vi "SInusoidy.vi"() -> ()   [LabVIEW 2020]
panel:
  in  "Amplituda 16":dbl
  in  "Faza 16":dbl
  in  "k 16":dbl
  in  "N 16":i32
  in  "Amplituda 15":dbl
  in  "Faza 15":dbl
  in  "k 15":dbl
  in  "N 15":i32
  out "Trzy osatatnie figury":cluster{"Array":dbl[], "Array":dbl[]}[](graph)
  in  "Amplituda 14":dbl
  in  "Faza 14":dbl
  in  "k 14":dbl
  in  "N 14":i32
  in  "Amplituda 13":dbl
  in  "Faza 13":dbl
  in  "k 13":dbl
  in  "N 13":i32
  in  "Amplituda 12":dbl
  in  "Faza 12":dbl
  in  "k 12":dbl
  in  "N 12":i32
  in  "Amplituda 11":dbl
  in  "Faza 11":dbl
  in  "k 11":dbl
  in  "N 11":i32
  in  "Amplituda 10":dbl
  in  "Faza 10":dbl
  in  "k 10":dbl
  in  "N 10":i32
  in  "Amplituda 9":dbl
  in  "Faza 9":dbl
  in  "k 9":dbl
  in  "N 9":i32
  in  "Amplituda 8":dbl
  in  "Faza 8":dbl
  in  "k 8":dbl
  in  "N 8":i32
  in  "Amplituda 7":dbl
  in  "Faza 7":dbl
  in  "k 7":dbl
  in  "N 7":i32
  out "Trzy pierwsze figury Lissajous":cluster{"Array":dbl[], "Array":dbl[]}[](graph)
  in  "Amplituda 6":dbl
  in  "Faza 6":dbl
  in  "k 6":dbl
  in  "N 6":i32
  in  "Amplituda 5":dbl
  in  "Faza 5":dbl
  in  "k 5":dbl
  in  "N 5":i32
  out "Dowolne figury Lissajous":cluster{"Y":dbl[], "Y":dbl[]}[](graph)
  in  "Amplituda 4":dbl
  in  "Faza 4":dbl
  in  "k 4":dbl
  in  "N 4":i32
  in  "Amplituda 3":dbl
  in  "Faza 3":dbl
  in  "k 3":dbl
  in  "N 3":i32
  in  "Amplituda 2":dbl
  in  "Faza 2":dbl
  in  "k 2":dbl
  in  "N 2":i32
  out "Do cosinusa":dbl[](graph)
  out "Do sinusa":dbl[](graph)
  in  "N":i32
  in  "Amplituda":dbl
  in  "Faza":dbl
  in  "k":dbl
  # "Pierwsza figura"
  # "Druga figura"
  # "Trzecia Figura"
  # "Do ostatnich figur"
  # "uno"
  # "duo"
  # "tres"
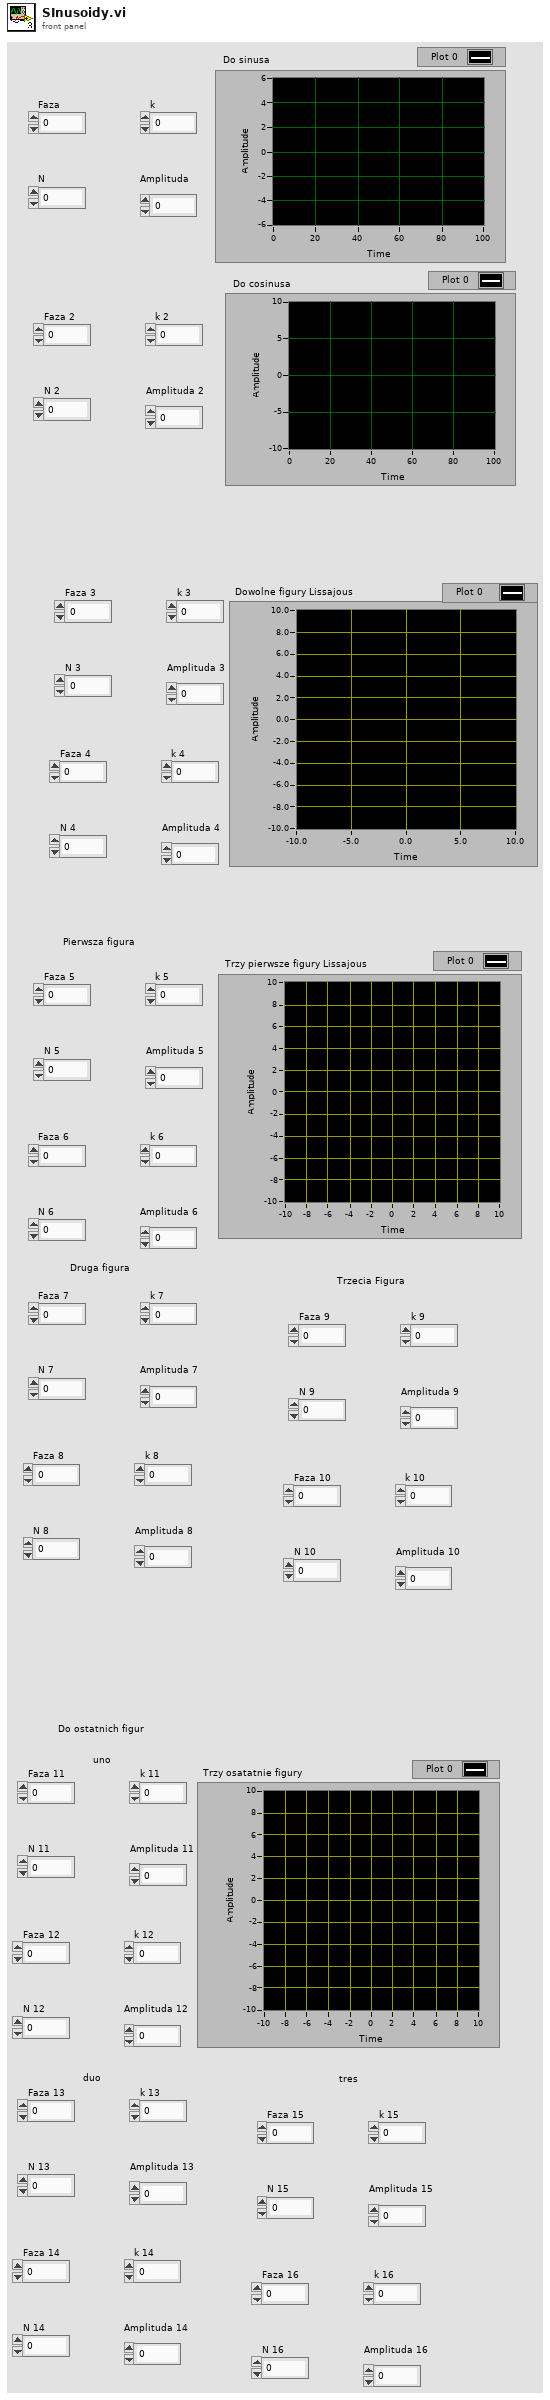
[diagram p1: front panel]
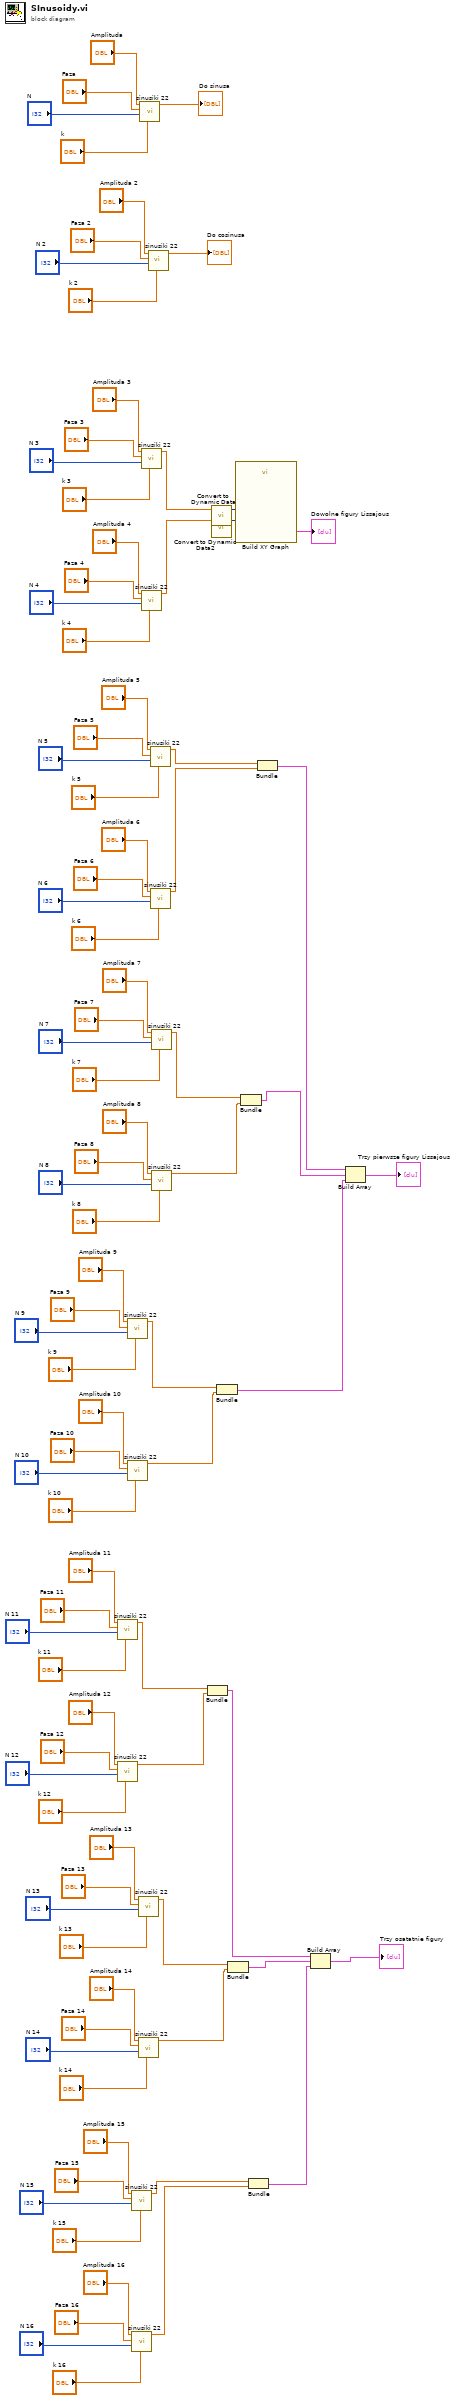
[diagram p0: block diagram]
diagram:
  n1 = call "sinusiki 22.vi"("k"="k 11", "N"="N 11", "Faza"="Faza 11", "Amplituda"="Amplituda 11") -> ("Array"=w26:dbl[])  [unwired: 7 in]
  n2 = call "sinusiki 22.vi"("k"="k 12", "N"="N 12", "Faza"="Faza 12", "Amplituda"="Amplituda 12") -> ("Array"=w25:dbl[])  [unwired: 7 in]
  n3 = call "sinusiki 22.vi"("k"="k 9", "N"="N 9", "Faza"="Faza 9", "Amplituda"="Amplituda 9") -> ("Array"=w38:dbl[])  [unwired: 7 in]
  n4 = call "sinusiki 22.vi"("k"="k 10", "N"="N 10", "Faza"="Faza 10", "Amplituda"="Amplituda 10") -> ("Array"=w37:dbl[])  [unwired: 7 in]
  n5 = call "sinusiki 22.vi"("k"="k 15", "N"="N 15", "Faza"="Faza 15", "Amplituda"="Amplituda 15") -> ("Array"=w3:dbl[])  [unwired: 7 in]
  n6 = call "sinusiki 22.vi"("k"="k 16", "N"="N 16", "Faza"="Faza 16", "Amplituda"="Amplituda 16") -> ("Array"=w2:dbl[])  [unwired: 7 in]
  n7 = call "sinusiki 22.vi"("k"="k 13", "N"="N 13", "Faza"="Faza 13", "Amplituda"="Amplituda 13") -> ("Array"=w16:dbl[])  [unwired: 7 in]
  n8 = call "sinusiki 22.vi"("k"="k 14", "N"="N 14", "Faza"="Faza 14", "Amplituda"="Amplituda 14") -> ("Array"=w15:dbl[])  [unwired: 7 in]
  n9 = call "sinusiki 22.vi"("k"="k", "N"="N", "Faza"="Faza", "Amplituda"="Amplituda") -> ("Array"=→"Do sinusa":dbl[])  [unwired: 7 in]
  n10 = call "sinusiki 22.vi"("k"="k 3", "N"="N 3", "Faza"="Faza 3", "Amplituda"="Amplituda 3") -> ("Array"=w72:dbl[])  [unwired: 7 in]
  n11 = call "sinusiki 22.vi"("k"="k 4", "N"="N 4", "Faza"="Faza 4", "Amplituda"="Amplituda 4") -> ("Array"=w70:dbl[])  [unwired: 7 in]
  n12 = call "sinusiki 22.vi"("k"="k 2", "N"="N 2", "Faza"="Faza 2", "Amplituda"="Amplituda 2") -> ("Array"=→"Do cosinusa":dbl[])  [unwired: 7 in]
  n13 = call "sinusiki 22.vi"("k"="k 5", "N"="N 5", "Faza"="Faza 5", "Amplituda"="Amplituda 5") -> ("Array"=w60:dbl[])  [unwired: 7 in]
  n14 = call "sinusiki 22.vi"("k"="k 6", "N"="N 6", "Faza"="Faza 6", "Amplituda"="Amplituda 6") -> ("Array"=w59:dbl[])  [unwired: 7 in]
  n15 = call "sinusiki 22.vi"("k"="k 7", "N"="N 7", "Faza"="Faza 7", "Amplituda"="Amplituda 7") -> ("Array"=w49:dbl[])  [unwired: 7 in]
  n16 = call "sinusiki 22.vi"("k"="k 8", "N"="N 8", "Faza"="Faza 8", "Amplituda"="Amplituda 8") -> ("Array"=w48:dbl[])  [unwired: 7 in]
  n17 = Bundle("Array"=w26, "Array"=w25) -> (w14:cluster{"Array":dbl[], "Array":dbl[]})  [unwired: 1 in]
  n18 = call "Convert to Dynamic Data"("Array"=w72) -> ("Dynamic Data Type"=w71:dynamicdata)  [unwired: 3 in]
  n19 = call "Convert to Dynamic Data2"("Array"=w70) -> ("Dynamic Data Type"=w69:dynamicdata)  [unwired: 3 in]
  n20 = Bundle("Array"=w38, "Array"=w37) -> (w35:cluster{"Array":dbl[], "Array":dbl[]})  [unwired: 1 in]
  n21 = Bundle("Array"=w16, "Array"=w15) -> (w13:cluster{"Array":dbl[], "Array":dbl[]})  [unwired: 1 in]
  n22 = call "Build XY Graph"("Y Input"=w69, "X Input"=w71) -> ("XY Graph"=→"Dowolne figury Lissajous":cluster{"X":dbl[], "Y":dbl[]}[])  [unwired: 8 in, 1 out]
  n23 = Bundle("Array"=w49, "Array"=w48) -> (w47:cluster{"Array":dbl[], "Array":dbl[]})  [unwired: 1 in]
  n24 = Bundle("Array"=w3, "Array"=w2) -> (w1:cluster{"Array":dbl[], "Array":dbl[]})  [unwired: 1 in]
  n25 = Bundle("Array"=w60, "Array"=w59) -> (w58:cluster{"Array":dbl[], "Array":dbl[]})  [unwired: 1 in]
  n26 = Build Array(w14, w13, w1) -> (→"Trzy osatatnie figury":cluster{"Array":dbl[], "Array":dbl[]}[])
  n27 = Build Array(w58, w47, w35) -> (→"Trzy pierwsze figury Lissajous":cluster{"Array":dbl[], "Array":dbl[]}[])
